vi "receiveData.vi"(8 "error in (no error)":errorcluster, 11 "Model in":refnum<class "Model.lvclass">) -> (0 "error out":errorcluster, 3 "Model out":refnum<class "Model.lvclass">)   [LabVIEW 2013, in "Model.lvclass"]
uses:
  Model.lvclass
  <userlib>/Common/ILC/ILC/ILC.lvclass
  <userlib>/Common/Devices/DistanceGauge/DistanceGauge/DistanceGauge.lvclass
  <userlib>/Common/Devices/ForceSensorCalculator/ForceSensorCalculator/ForceSensorCalculator.lvclass
  <userlib>/Common/ILC/Typedefs/LimitSwitches.ctl
  <userlib>/Common/ILC/Typedefs/ILCTypedefs.lvlib
  Typedefs/ForceDemand.ctl
  Typedefs/M2AADTTypedefs.lvlib
  <userlib>/Common/Devices/DistanceGauge/Typedefs/Distance Data.ctl
  <userlib>/Common/Devices/DistanceGauge/DistanceGauge.lvlib
  Typedefs/InputData.ctl
  UserEvents/UserEvents.lvclass
  ApplicationElements/Thermocouple/Thermocouple.lvclass
  Typedefs/ThermocoupleData.ctl
  ApplicationElements/Log/TestDataLog/TestDataLog.lvclass
  <userlib>/Common/Devices/EncoderConverter/EncoderConverter/EncoderConverter.lvclass
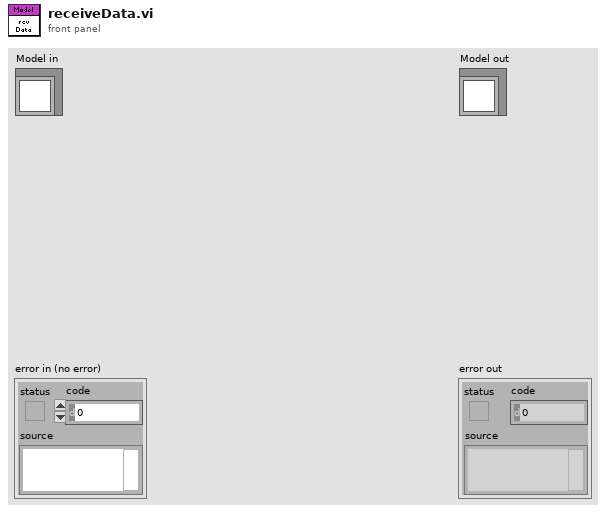
[diagram p1: front panel]
types:
  T1 = typedef "M2AADTTypedefs.lvlib/ThermocoupleData.ctl" = cluster{"Motor Temperature":dbl[unit]}
  T2 = typedef "M2AADTTypedefs.lvlib/InputData.ctl" = cluster{"Limit Switches":T3, "SSI Encoder":i32, "Force Measured":T4, "Distance Data":T5, "Thermocouple Data":T1}
  T3 = typedef "ILCCommon.lvlib/ILCTypedefs.lvlib/LimitSwitches.ctl" = cluster{"1":bool, "2":bool}
  T4 = typedef "M2AADTTypedefs.lvlib/ForceDemand.ctl" = dbl[unit]
  T5 = typedef "DistanceGauge.lvlib/Distance Data.ctl" = cluster{"Distance Measured 1":dbl[unit], "Distance Measured 2":dbl[unit]}
  T6 = typedef "M2AADTTypedefs.lvlib/PubDataEvents.ctl" = cluster{"State":refnum<user-event>, "ErrorCode":refnum<user-event>, "OutputData":refnum<user-event>, "InputData":refnum<user-event>, "ControllerData":refnum<user-event>, "TestStatus":refnum<user-event>, "LogPath":refnum<user-event>, "StiffnessData":refnum<user-event>}
  T7 = typedef "ILCCommon.lvlib/ILCTypedefs.lvlib/ADCsInEngineeringUnits.ctl" = cluster{"Ch1":dbl[unit], "Ch2":dbl[unit], "Ch3":dbl[unit], "Ch4":dbl[unit]}
  T8 = typedef "ILCCommon.lvlib/ILCTypedefs.lvlib/InputData.ctl" = cluster{"Input Channels":T9, "Limit Switches":T3, "Tachometer":u16, "SSI Encoder":i32, "ADCs":T10}
  T9 = typedef "ILCCommon.lvlib/ILCConfiguration.lvlib/InputChannels.ctl" = enum16{"Channel 0", "3 Channels", "5 Channels"}
  T10 = typedef "ILCCommon.lvlib/ILCTypedefs.lvlib/ADCs.ctl" = cluster{"Ch0":i32, "Ch1":i32, "Ch2":i32, "Ch3":i32, "Ch4":i32}
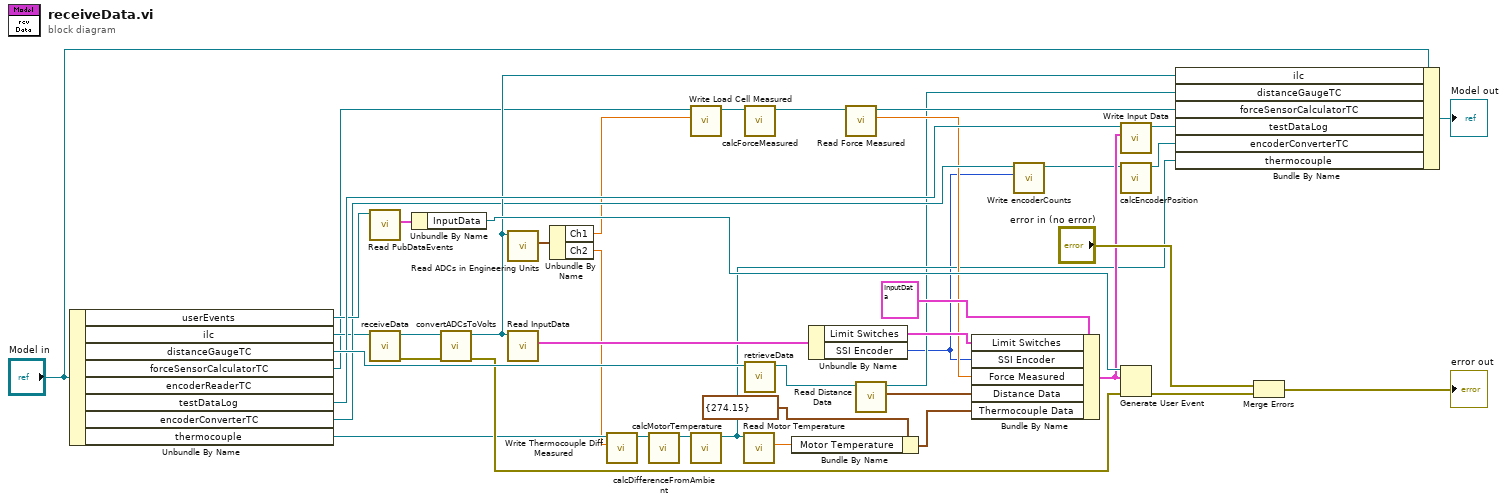
[diagram p0: block diagram]
diagram:
  n1 = Unbundle By Name("Model in") -> ("userEvents"=w24:refnum<class "UserEvents.lvclass">, "ilc"=w17:refnum<class "ILC.lvclass">, "distanceGaugeTC"=w40:refnum<class "DistanceGaugeTC.lvclass">, "forceSensorCalculatorTC"=w14:refnum<class "ForceSensorCalculatorTC.lvclass">, "testDataLog"=w27:refnum<class "TestDataLog.lvclass">, "encoderConverterTC"=w21:refnum<class "EncoderConverterTC.lvclass">, "thermocouple"=w13:refnum<class "Thermocouple.lvclass">)  [unwired: 1 out]
  n2 = call "Read PubDataEvents.vi"("UserEvents in"=w24) -> ("PubDataEvents"=w18:T6)  [unwired: 9 in, 1 out]
  n3 = call <userlib>:"receiveData.vi"("ILC in"=w17) -> ("error out"=w35:errorcluster, "ILC out"=w36:refnum<class "ILC.lvclass">)  [unwired: 9 in]
  n4 = Unbundle By Name(w18) -> ("InputData"=w25:refnum<user-event>)
  n5 = call <userlib>:"convertADCsToVolts.vi"("error in (no error)"=w35, "ILC in"=w36) -> ("error out"=w34:errorcluster, "ILC out"=w23:refnum<class "ILC.lvclass">)  [unwired: 8 in]
  n6 = call <userlib>:"Read ADCs in Engineering Units.vi"("ILC in"=w23) -> ("ADCs in Engineering Units"=w33:T7)  [unwired: 9 in, 1 out]
  n7 = call <userlib>:"Read InputData.vi"("ILC in"=w23) -> ("InputData"=w29:T8)  [unwired: 9 in, 1 out]
  n8 = Unbundle By Name(w33) -> ("Ch1"=w16:dbl[unit], "Ch2"=w11:dbl[unit])
  n9 = call "Write Thermocouple Diff Measured.vi"("Thermocouple Diff Measured"=w11, "Thermocouple in"=w13) -> ("Thermocouple out"=w12:refnum<class "Thermocouple.lvclass">)  [unwired: 9 in]
  n10 = call "calcDifferenceFromAmbient.vi"("Thermocouple in"=w12) -> ("Thermocouple out"=w8:refnum<class "Thermocouple.lvclass">)  [unwired: 9 in, 1 out]
  n11 = call <userlib>:"Write Load Cell Measured.vi"("Load Cell Measured"=w16, "ForceSensor in"=w14) -> ("ForceSensor out"=w15:refnum<class "ForceSensorCalculatorTC.lvclass">)  [unwired: 9 in]
  n12 = call "calcMotorTemperature.vi"("Thermocouple in"=w8) -> ("Thermocouple out"=w7:refnum<class "Thermocouple.lvclass">)  [unwired: 9 in, 1 out]
  n13 = call "Read Motor Temperature.vi"("Thermocouple in"=w7) -> ("Motor Temperature"=w6:dbl[unit])  [unwired: 9 in, 1 out]
  n14 = call <userlib>:"calcForceMeasured.vi"("ForceSensor in"=w15) -> ("ForceSensor out"=w32:refnum<class "ForceSensorCalculatorTC.lvclass">)  [unwired: 9 in, 1 out]
  n15 = call <userlib>:"retrieveData.vi"("DistanceGauge in"=w40) -> ("DistanceGauge out"=w5:refnum<class "DistanceGaugeTC.lvclass">)  [unwired: 8 in, 2 out]
  n16 = Bundle By Name(cluster=T1 {"Motor Temperature"=274.15} ("Thermocouple Data"), "Motor Temperature"=w6) -> (w9:T1)
  n17 = Unbundle By Name(w29) -> ("Limit Switches"=w28:T3, "SSI Encoder"=w1:i32)
  n18 = call <userlib>:"Read Force Measured.vi"("ForceSensor in"=w32) -> ("Force Demand"=w19:dbl[unit], "ForceSensor out"=w31:refnum<class "ForceSensorCalculatorTC.lvclass">)  [unwired: 9 in]
  n19 = call <userlib>:"Read Distance Data.vi"("DistanceGauge in"=w5) -> ("Distance Data"=w3:T5, "DistanceGauge out"=w4:refnum<class "DistanceGaugeTC.lvclass">)  [unwired: 9 in]
  n20 = Bundle By Name(cluster=T2 {"Limit Switches"={"1"=FALSE, "2"=FALSE}, "SSI Encoder"=0, "Force Measured"=0.0, "Distance Data"={"Distance Measured 1"=1.0, "Distance Measured 2"=1.0}, "Thermocouple Data"={"Motor Temperature"=274.15}} ("event data"), "Limit Switches"=w28, "SSI Encoder"=w1, "Force Measured"=w19, "Distance Data"=w3, "Thermocouple Data"=w9) -> (w22:T2)
  n21 = call <userlib>:"Write encoderCounts.vi"("encoderCounts"=w1, "EnccoderConverter in"=w21) -> ("EnccoderConverter out"=w20:refnum<class "EncoderConverterTC.lvclass">)  [unwired: 9 in]
  n22 = call "Write Input Data.vi"("Input Data"=w22, "Logger in"=w27) -> ("Logger out"=w26:refnum<class "TestDataLog.lvclass">)  [unwired: 9 in]
  n23 = call <userlib>:"calcEncoderPosition.vi"("EnccoderConverter in"=w20) -> ("EnccoderConverter out"=w2:refnum<class "EncoderConverterTC.lvclass">)  [unwired: 9 in, 1 out]
  n24 = Generate User Event(user event=w25, event data cluster=w22, error in=w34) -> (error out=w38:errorcluster)  [unwired: 1 in, 1 out]
  n25 = Bundle By Name(cluster="Model in", "ilc"=w23, "distanceGaugeTC"=w4, "forceSensorCalculatorTC"=w31, "testDataLog"=w26, "encoderConverterTC"=w2, "thermocouple"=w7) -> (→"Model out":refnum<class "Model.lvclass">)
  n26 = Merge Errors("error in (no error)", w38) -> (→"error out":errorcluster)
